vi "stepper controller.vi"(7 "stepper motor action":T2, 8 "set":dbl format="%#_13g", 9 "stepper motor state":T1) -> (1 "stepper motor state OUT":T1)   [LabVIEW 2018]
uses:
  stepper motor state.ctl
  stepper motor action.ctl
  internal stepper state.ctl
panel:
  in  "VISA session":refnum<visa-resource-name>="GPIB0::25::INSTR"
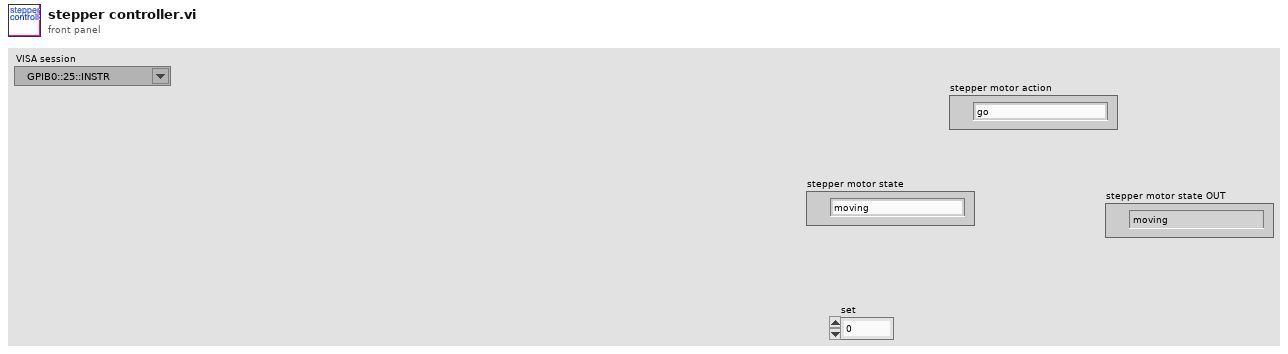
[diagram p1: front panel]
types:
  T1 = typedef "stepper motor state.ctl" = enum16{"moving", "stopped"}
  T2 = typedef "stepper motor action.ctl" = enum16{"go", "stop", "check", "init", "sync", "set"}
  T3 = cluster{"initialized?":bool, "VISA session":refnum<visa-resource-name>}
  T4 = typedef "internal stepper state.ctl" = cluster{"initialized?":bool, "VISA address":refnum<visa-resource-name>}
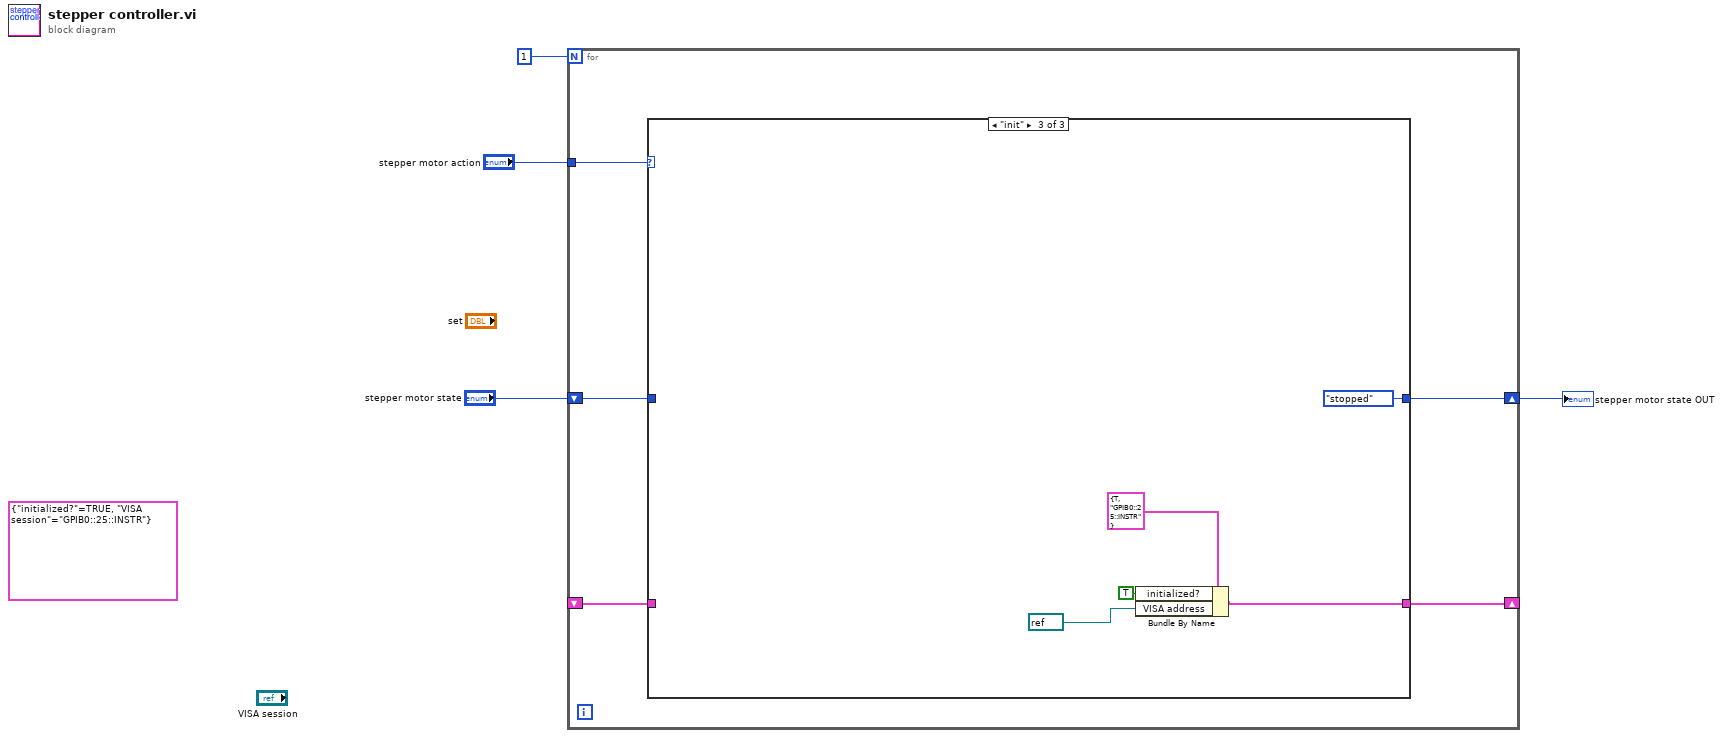
[diagram p0: block diagram]
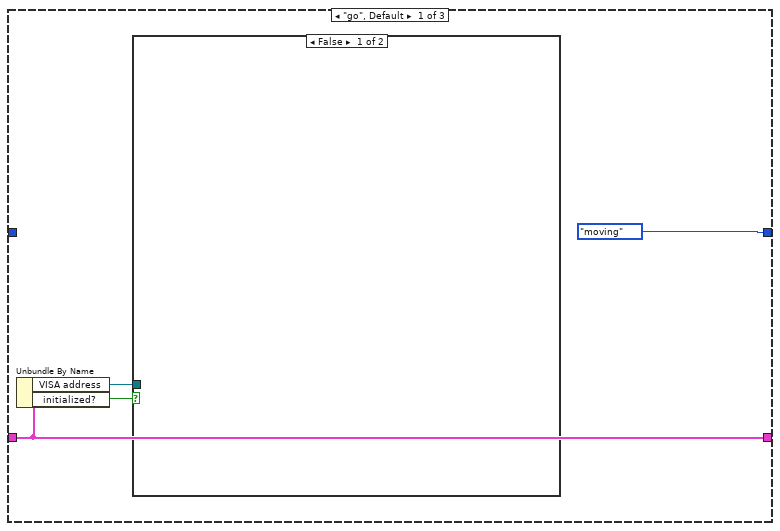
[diagram p2: hidden frame]
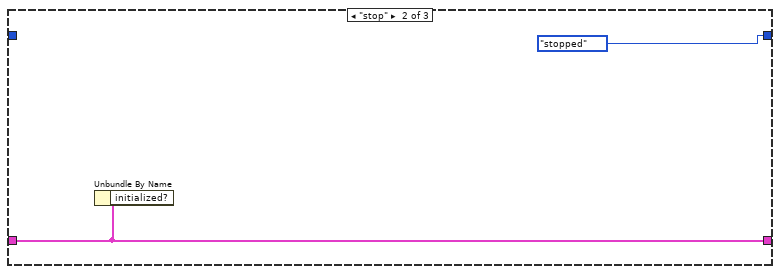
[diagram p4: hidden frame]
diagram:
  (unwired) T3 {"initialized?"=TRUE, "VISA session"="GPIB0::25::INSTR"}
  n1 = for {
    N: 1 -> [_]
    tunnel: "stepper motor action" -> [w9]
    shift-right: [w8] -> w3
    shift-left: "stepper motor state" -> [w7]
    shift-right: [w6] -> _
    shift-left: _ -> [w5]
    n2 = case shown="\"init\"" w9 {
      tunnel: w7 -> [_ _ _]
      tunnel: [stepper_motor_state."moving" ("stepper motor state") stepper_motor_state."stopped" ("stepper motor state") stepper_motor_state."stopped" ("stepper motor state")] -> w8
      tunnel: [w12 w14 w19] -> w6
      tunnel: w5 -> [w12 w14 _]
      frame "go", Default {
        n3 = Unbundle By Name(w12) -> ("VISA address"=w10:refnum<visa-resource-name>, "initialized?"=w11:bool)
        n4 = case shown="False" w11 {
          tunnel: w10 -> [_ _]
          frame False {
          }
          frame True {
          }
        }
      }
      frame "stop" {
        n5 = Unbundle By Name(w14) -> ()  [unwired: 1 out]
      }
      frame "init" {
        n6 = Bundle By Name(cluster=T4 {"initialized?"=TRUE, "VISA address"="GPIB0::25::INSTR"} ("internal stepper state"), "initialized?"=TRUE, "VISA address"=refnum<visa-resource-name> refnum ("VISA session")) -> (w19:T4)
      }
    }
  }
  "stepper motor state OUT" <- w3
